vi "Read Key (Double).vi"(7 "section":string, 8 "error in (no error)":errorcluster, 9 "default value":dbl, 10 "key":string, 11 "refnum":T1) -> (0 "error out":errorcluster, 1 "value":dbl, 2 "found?":bool, 3 "refnum out":T1)   [LabVIEW 2020, in "NI_LVConfig.lvlib"]
doc: "Reads a value associated with a key in a specified section from the configuration data identified by <B>refnum</B>. If the key does not exist, the VI returns the default value. This VI supports multibyte characters in strings. Wire data to the <B>default value</B> input to determine the polymorphic instance to use or manually select the instance."
uses:
  NI_LVConfig.lvlib
  Config Data RefNum.ctl
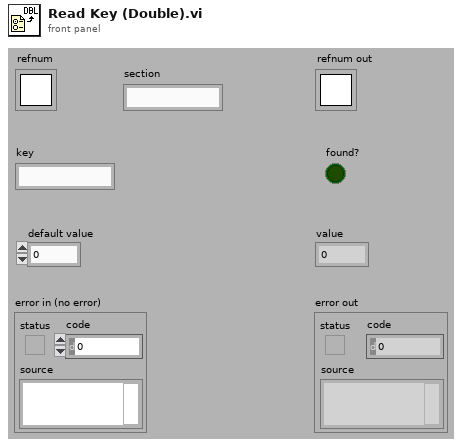
[diagram p1: front panel]
types:
  T1 = typedef "NI_LVConfig.lvlib/Config Data RefNum.ctl" = refnum<k1>
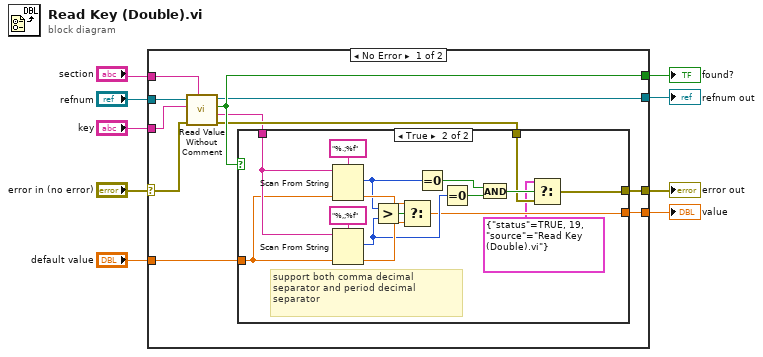
[diagram p0: block diagram]
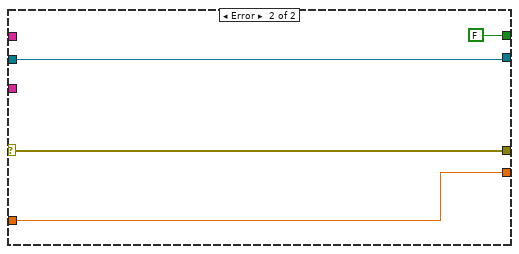
[diagram p3: hidden frame]
diagram:
  n1 = case shown="No Error" "error in (no error)" {
    selector: "error in (no error)" -> [w13 w42]
    tunnel: [w19 w42] -> w8
    tunnel: [w15 w39] -> w1
    tunnel: "section" -> [w12 _]
    tunnel: "key" -> [w11 _]
    tunnel: "default value" -> [w20 w41]
    tunnel: [w17 FALSE ("key exists?")] -> w4
    tunnel: [w18 w41] -> w3
    tunnel: "refnum" -> [w10 w39]
    frame No Error {
      n2 = call "Read Value Without Comment.vi"("section"=w12, "error in (no error)"=w13, "key"=w11, "refnum"=w10) -> ("error out"=w16:errorcluster, "value"=w14:string, "found?"=w17:bool, "refnum out"=w15:T1)  [unwired: 4 out]
      n3 = case shown="True" w17 {
        tunnel: w14 -> [_ w36]
        tunnel: w20 -> [w21 w23]
        tunnel: [w21 w28] -> w18
        tunnel: w16 -> [w22 w26]
        tunnel: [w22 w24] -> w19
        frame False {
        }
        frame True {
          # "support both comma decimal separator and period decimal separator"
          n4 = Scan From String(format string="%.;%f" ("Format String"), input string=w36, default 1=w23) -> (offset past scan=w32:u32, output 1=w34:dbl)  [unwired: 2 in, 2 out]
          n5 = Scan From String(format string="%,;%f" ("Format String"), input string=w36, default 1=w23) -> (offset past scan=w30:u32, output 1=w33:dbl)  [unwired: 2 in, 2 out]
          n6 = Greater?(x=w32, y=w30) -> (0:w35:bool)
          n7 = Select(t=w34, s=w35, f=w33) -> (s? t:f=w28:dbl)
          n8 = Equal To 0?(x=w32) -> (x = 0?=w31:bool)
          n9 = Equal To 0?(x=w30) -> (x = 0?=w29:bool)
          n10 = And(x=w31, y=w29) -> (x .and. y?=w27:bool)
          n11 = Select(t=cluster{"status":bool, u16, "source":string} {"status"=TRUE, 19, "source"="Read Key (Double).vi"} ("f"), s=w27, f=w26) -> (s? t:f=w24:errorcluster)
        }
      }
    }
    frame Error {
    }
  }
  "error out" <- w8
  "found?" <- w4
  "value" <- w3
  "refnum out" <- w1
